vi "Failure Message.vi"() -> ()   [LabVIEW 2017, in "Transparent Assertions.Tests.lvlib" / "Assert Not Error Code.lvlib"]
uses:
  Assert Not Error Code.lvlib
  src/Transparent Assertions/Transparent Assertions.lvlib
panel:
  out "error out":errorcluster
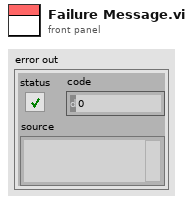
[diagram p1: front panel]
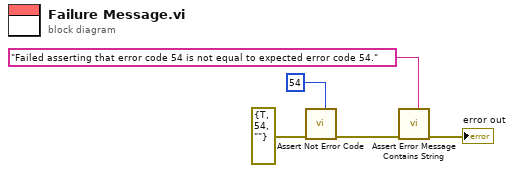
[diagram p0: block diagram]
diagram:
  n1 = call "Assert Not Error Code.vi"("Expected"=54, "error in (no error)"=errorcluster {"status"=TRUE, "code"=54, "source"=""}) -> ("error out"=w3:errorcluster)  [unwired: 9 in]
  n2 = call "Assert Error Message Contains String.vi"("Expected"="Failed asserting that error code 54 is not equal to expected error code 54." ("Message (\"\")"), "error in (no error)"=w3) -> ("error out"=→"error out":errorcluster)  [unwired: 9 in]
